vi "Get Control Portion Image.vi"(8 "error in (no error)":errorcluster, 11 "Ctl Ref":refnum<vi>) -> (0 "error out":errorcluster, 2 "Control Image":T1, 3 "Ctl Ref out":refnum<vi>)   [LabVIEW 2020, in "MacroAssert.lvlib"]
doc: "Gets the image of the control identified by <B>Ctl Ref</B>."
uses:
  MacroAssert.lvlib
  <vilib>/picture/picture.llb/imagedata.ctl
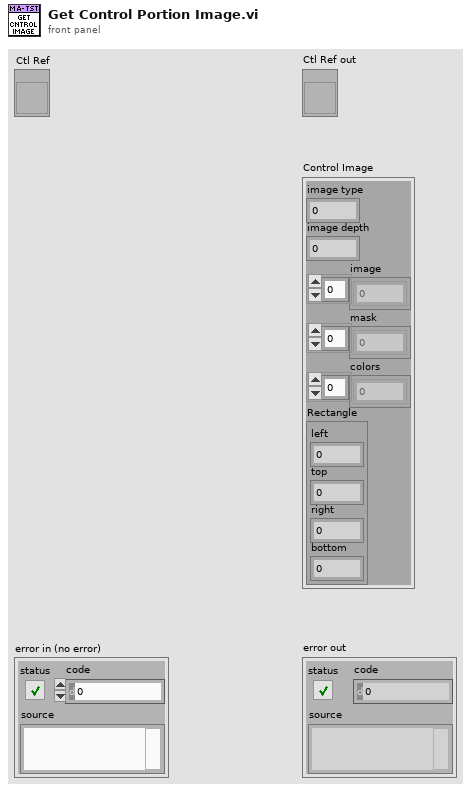
[diagram p1: front panel]
types:
  T1 = typedef "imagedata.ctl" = cluster{"image type":i32, "image depth":i32, "image":u8[], "mask":u8[], "colors":u32[], "Rectangle":cluster{"left":i16, "top":i16, "right":i16, "bottom":i16}}
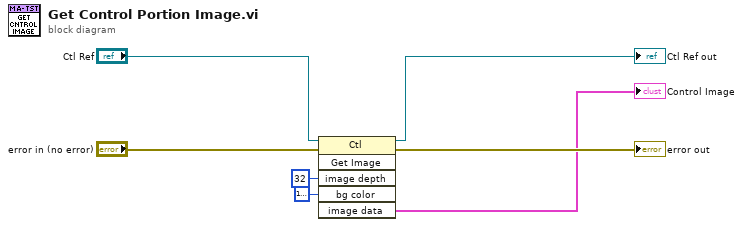
[diagram p0: block diagram]
diagram:
  n1 = invoke class="Ctl" method="Get Image"(reference="Ctl Ref", error in="error in (no error)", "image depth"=32 ("Image Depth"), "bg color"=u32 16777238 ("Background Color")) -> (reference out=→"Ctl Ref out":refnum<vi>, error out=→"error out":errorcluster, "image data"=→"Control Image":T1)  [unwired: 2 in, 3 out]
